vi "TriggerPosPID.vi"(5 "I":dbl format="%#_13g", 6 "D":dbl=10.0 format="%#_13g", 7 "P":dbl=0.3 format="%#_13g", 8 "error in":errorcluster, 10 "Button Input":bool, 11 "CAN Talon SRX Ref":T1={"DeviceStatus"={"status"=FALSE, "code"=0, "source"=""}, "Type"=enum."PWM", "PWM"={"PWM Channel"=enum."PWM 1", "DeadBand"={"Name"="", "maxPositivePwm"=0, "minPositivePwm"=0, "centerPwm"=0, "maxNegativePwm"=0, "minNegativePwm"=0, "angularRange"=0}}, "CAN"={"Device Number"=0, "Control Mode"=enum."Percent VBus", "Semaphore"=refnum, "Max Vout"=12.0, "TalonSRX Control Mode"=enum."Percent VBus"}, "Invert"=FALSE}) -> (0 "error out":errorcluster)   [LabVIEW 2015]
uses:
  <vilib>/Rock Robotics/WPI/MotorControl/WPI_MotorControlDeviceRef.ctl
  <vilib>/Rock Robotics/WPI/MotorControl/WPI_MotorControlType.ctl
  <vilib>/Rock Robotics/SystemInterfaces/DIO/FPGA_DIOPWMChannel.ctl
  <vilib>/Rock Robotics/WPI/PWM/WPI_PWMDeadband.ctl
  <vilib>/Rock Robotics/WPI/CAN/Jaguar/SubVIs/WPI_CANJaguar_ControlMode.ctl
  <vilib>/Rock Robotics/WPI/CAN/TalonSRX/WPI_CANTalonSRX_APIControlMode.ctl
panel:
  in  "Joystick Throttle":dbl
  out "To Motor Output":dbl
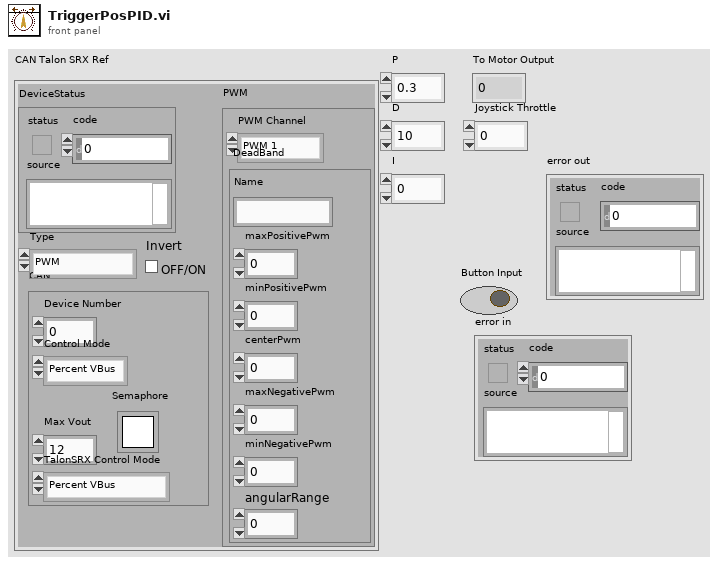
[diagram p1: front panel]
types:
  T1 = typedef "WPI_MotorControlDeviceRef.ctl" = cluster{"DeviceStatus":errorcluster, "Type":T2, "PWM":cluster{"PWM Channel":T3, "DeadBand":T4}, "CAN":cluster{"Device Number":u8, "Control Mode":T5, "Semaphore":T6, "Max Vout":dbl, "TalonSRX Control Mode":T7}, "Invert":bool}
  T2 = typedef "WPI_MotorControlType.ctl" = enum16{"PWM", "CAN", "CANTalonSRX"}
  T3 = typedef "FPGA_DIOPWMChannel.ctl" = enum8{"PWM 0", "PWM 1", "PWM 2", "PWM 3", "PWM 4", "PWM 5", "PWM 6", "PWM 7", "PWM 8", "PWM 9", "PWM MXP 0", "PWM MXP 1", "PWM MXP 2", "PWM MXP 3", "PWM MXP 4", "PWM MXP 5", "PWM MXP 6", "PWM MXP 7", "PWM MXP 8", "PWM MXP 9", "Invalid"}
  T4 = typedef "WPI_PWMDeadband.ctl" = cluster{"Name":string, "maxPositivePwm":i32, "minPositivePwm":i32, "centerPwm":i32, "maxNegativePwm":i32, "minNegativePwm":i32, "angularRange":u16}
  T5 = typedef "WPI_CANJaguar_ControlMode.ctl" = enum8{"Percent VBus", "Current", "Speed", "Position", "Voltage"}
  T6 = typedef "Semaphore RefNum" = refnum<k1>
  T7 = typedef "WPI_CANTalonSRX_APIControlMode.ctl" = enum8{"Percent VBus", "Speed", "Position", "Slave", "Unchanged / Invalid", "Voltage Compensation", "Current", "Motion Profile"}
  T8 = typedef "WPI_CANTalonSRX_GlobalStatus.ctl" = cluster{"Applied Throttle":dbl, "Module Enabled":bool, "CAN Error":errorcluster, "Closed Loop Error":dbl, "Forward Limit Switch Closed":bool, "Reverse Limit Switch Closed":bool, "Sensor Position":dbl, "Sensor Velocity":dbl, "Current":dbl, "Sticky Fault - Over Temp":bool, "Sticky Fault - Under Voltage":bool, "Sticky Fault - Forward Limit":bool, "Sticky Fault - Reverse Limit":bool, "Sticky Fault - Forward Soft Limit":bool, "Sticky Fault - Reverse Soft Limit":bool, "Brake is Enabled":bool, "Encoder Position":dbl, "Encoder Velocity":dbl, "Encoder Index Count":dbl, "Encoder A Pin State":bool, "Encoder B Pin State":bool, "Encoder Index Pin State":bool, "Analog In":dbl, "Analog In Velocity":dbl, "Temperature (C)":dbl, "Battery Voltage":dbl, "Control 5 Is Supported":bool, "Current Profile Slot Select":dbl, "Pos Div 8":bool, "Vel Div 4":bool, "Pulse Width Position":i32, "Pulse Width Velocity":i32, "Pulse Width Rise To Rise (us)":i32, "Pulse Width Rise To Fall (us)":i32, "Mot Prof Active Is Under Run":bool, "Mot Prof Active Has Under Run":bool, "Mot Prof Active Is Last":bool, "Mot Prof Active Velocity Only":bool, "Mot Prof Active Is Valid":bool, "Mot Prof Buffer Is Full":bool, "Mot Prof Active Profile Slot Select":i32, "Mot Prof NextID":i32, "Mot Prof Count":i32, "Mot Prof Active Velocity":dbl, "Mot Prof Active Position":dbl, "Mot Prof Output Enable":i32}
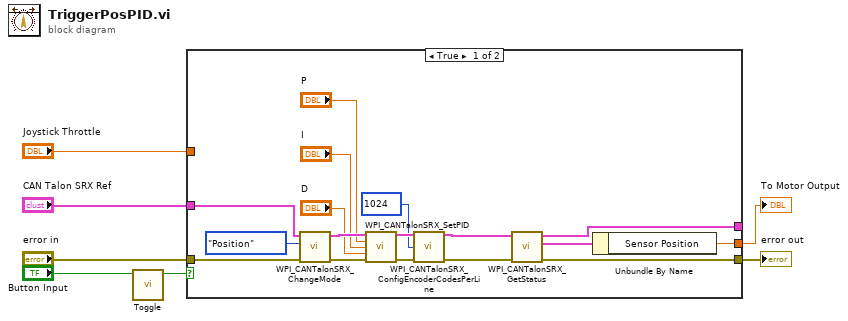
[diagram p0: block diagram]
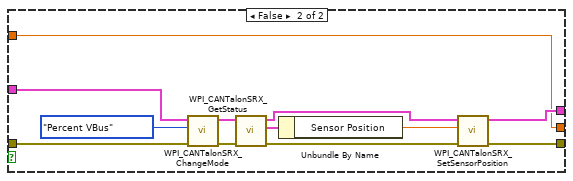
[diagram p2: hidden frame]
diagram:
  n1 = call "Toggle.vi"("Button Input"="Button Input") -> ("Toggle Output"=w6:bool)  [unwired: 9 in, 1 out]
  n2 = case shown="True" w6 {
    tunnel: [w20 w34] -> _
    tunnel: [w23 w27] -> w4
    tunnel: "CAN Talon SRX Ref" -> [w22 w31]
    tunnel: "Joystick Throttle" -> [_ w27]
    tunnel: [w8 w26] -> w2
    tunnel: "error in" -> [w9 w25]
    frame True {
      n3 = call <vilib>:"WPI_CANTalonSRX_ChangeMode.vi"("error in (no error)"=w9, "Control Mode"=WPI_CANTalonSRX_APIControlMode."Position", "CAN Talon SRX Ref"=w22) -> ("error out"=w18:errorcluster, "CAN Talon SRX Ref"=w19:T1)  [unwired: 7 in]
      n4 = call <vilib>:"WPI_CANTalonSRX_SetPID.vi"("CAN Talon SRX Ref"=w19, "P"="P", "I"="I", "D"="D", "error in (no error)"=w18) -> ("CAN Talon SRX Ref"=w14:T1, "error out"=w11:errorcluster)  [unwired: 9 in]
      n5 = call <vilib>:"WPI_CANTalonSRX_ConfigEncoderCodesPerLine.vi"("CAN Talon SRX Ref"=w14, "Number Encoder Lines\n(Counts Per Rotation)"=u32 1024 ("Number Encoder Lines\n(Counts Per Rotation)"), "error in (no error)"=w11) -> ("CAN Talon SRX Ref"=w13:T1, "error out"=w10:errorcluster)  [unwired: 11 in]
      n6 = call <vilib>:"WPI_CANTalonSRX_GetStatus.vi"("error in (no error)"=w10, "CAN Talon SRX Ref"=w13) -> ("error out"=w8:errorcluster, "Talon SRX Status"=w24:T8, "CAN Talon SRX Ref"=w20:T1)  [unwired: 7 in]
      n7 = Unbundle By Name(w24) -> ("Sensor Position"=w23:dbl)
    }
    frame False {
      n8 = call <vilib>:"WPI_CANTalonSRX_ChangeMode.vi"("error in (no error)"=w25, "Control Mode"=WPI_CANTalonSRX_APIControlMode."Percent VBus", "CAN Talon SRX Ref"=w31) -> ("error out"=w29:errorcluster, "CAN Talon SRX Ref"=w32:T1)  [unwired: 7 in]
      n9 = call <vilib>:"WPI_CANTalonSRX_GetStatus.vi"("error in (no error)"=w29, "CAN Talon SRX Ref"=w32) -> ("error out"=w28:errorcluster, "Talon SRX Status"=w36:T8, "CAN Talon SRX Ref"=w35:T1)  [unwired: 7 in]
      n10 = Unbundle By Name(w36) -> ("Sensor Position"=w33:dbl)
      n11 = call <vilib>:"WPI_CANTalonSRX_SetSensorPosition.vi"("error in (no error)"=w28, "New Sensor Position"=w33, "CAN Talon SRX Ref"=w35) -> ("error out"=w26:errorcluster, "CAN Talon SRX Ref"=w34:T1)  [unwired: 7 in]
    }
  }
  "To Motor Output" <- w4
  "error out" <- w2
